vi "0000_Initialize.vi"(8 "error in (no error)":errorcluster, 9 "Slot Settings":T1, 11 "0000 in":refnum<class "Module Template.lvclass">) -> (0 "error out":errorcluster, 3 "0000 out":refnum<class "Module Template.lvclass">)   [LabVIEW 2017, in "Modules.lvlib" / "Module Template.lvclass"]
uses:
  Module Template.lvclass
  RSI Module/Slot Settings.ctl
  C:/Users/dbuck/Documents/GitHub/Scan-Engine-Custom-Device-Classes/Source/RSI Module/RSI Module.lvclass
  RSI Module/Channels.ctl
  RSI Module/Channel Type.ctl
  RSI Module/Module Models.ctl
  Module Template.lvclass/Module Template.ctl
  RSI Module/RSI Module.lvclass
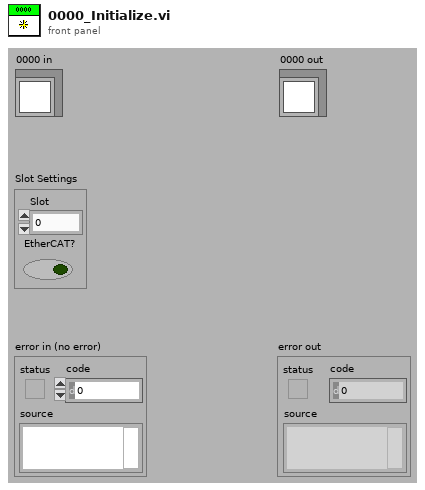
[diagram p1: front panel]
types:
  T1 = typedef "Modules.lvlib/RSI Module.lvclass/Slot Settings.ctl" = cluster{"Slot":u32, "EtherCAT?":bool}
  T2 = typedef "Modules.lvlib/RSI Module.lvclass/Module Models.ctl" = enum16{"Empty", "NI 9201", "NI 9203", "NI 9205", "NI 9206", "NI 9207", "NI 9208", "NI 9211", "NI 9212", "NI 9213", "NI 9214", "NI 9215", "NI 9217", "NI 9219", "NI 9220", "NI 9221", "NI 9222", "NI 9223", "NI 9225", "NI 9227", "NI 9229", "NI 9233", "NI 9234", "NI 9235", "NI 9236", "NI 9237", "NI 9239", "NI 9242", "NI 9244", "NI 9263", "NI 9264", "NI 9265", "NI 9269", "NI 9375", "NI 9401", "NI 9402", "NI 9403", "NI 9411", "NI 9421", "NI 9422", "NI 9423", "NI 9425", "NI 9426", "NI 9435", "NI 9437", "NI 9472", "NI 9474", "NI 9475", "NI 9476", "NI 9477", "NI 9478", "NI 9481", "NI 9482", "NI 9485"}
  T3 = typedef "Modules.lvlib/RSI Module.lvclass/Channels.ctl" = cluster{"# Input Channels":i32, "# Output Channels":i32, "Channel Type":T4, "Units":string}
  T4 = typedef "Modules.lvlib/RSI Module.lvclass/Channel Type.ctl" = enum16{"Analog", "Digital"}
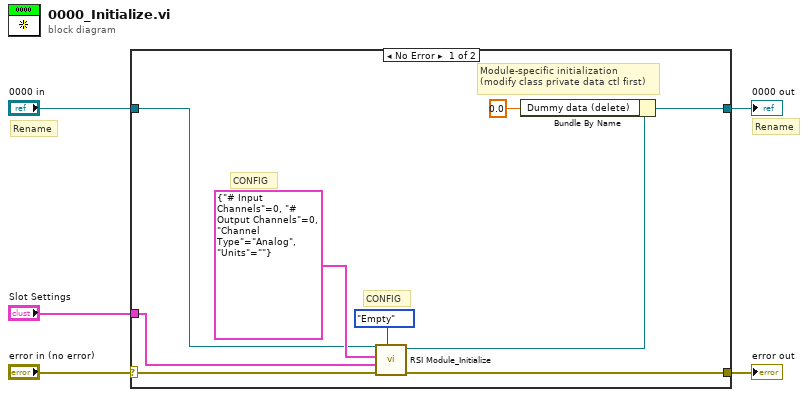
[diagram p0: block diagram]
diagram:
  # "Rename"
  # "Rename"
  n1 = case shown="No Error" "error in (no error)" {
    selector: "error in (no error)" -> [w11 w16]
    tunnel: [w10 w16] -> w4
    tunnel: [w8 w15] -> w2
    tunnel: "0000 in" -> [w13 w15]
    tunnel: "Slot Settings" -> [w12 _]
    frame No Error {
      # "Module-specific initialization\n(modify class private data ctl first)"
      # "CONFIG"
      # "CONFIG"
      n2 = call "RSI Module_Initialize.vi"("Module Model"=Module_Models."Empty", "error in (no error)"=w11, "Slot Settings"=w12, "Channels"=T3 {"# Input Channels"=0, "# Output Channels"=0, "Channel Type"=enum."Analog", "Units"=""}, "RSI Module in"=w13) -> ("error out"=w10:errorcluster, "RSI Module out"=w9:refnum<class "Module Template.lvclass">)  [unwired: 5 in]
      n3 = Bundle By Name(cluster=w9, "Dummy data (delete)"=0.0 ("Dummy Data")) -> (w8:refnum<class "Module Template.lvclass">)
    }
    frame Error {
    }
  }
  "error out" <- w4
  "0000 out" <- w2
